vi "Set TimeToPlot.vi"(8 "error in (no error)":errorcluster, 10 "Time to Plot":dbl=1800.0 format="%<%H:%M:%S>t", 11 "BluePlotHandle in":refnum<class "RocketPlotHandle.lvclass">) -> (0 "error out":errorcluster, 3 "BluePlotHandle out":refnum<class "RocketPlotHandle.lvclass">)   [LabVIEW 2021, in "RocketPlotHandle.lvclass"]
doc: "Load plot configuration into the attached plot instance.\n\nNote that this will load ALL plot settings from the input \"plot config\" cluster input.\nThere is no mechanism for specifying only a subset of these settings to be loaded.\nIt's all or nothin'\n\nIf you ever needed to modify/load only 1 aspect of a plot, then I recommend:\n- perform \"get plot config\"\n- perform in-place modification of the plot config cluster to adjust what you want to specifically change\n- perform \"load plot config\""
uses:
  RocketPlotHandle.lvclass
  RocketPlotHandle.lvclass/RocketPlotHandle.ctl
  TypeDefs/plot handle queue data.ctl
  TypeDefs/Plot QSM action.ctl
  RocketPlot.lvlib
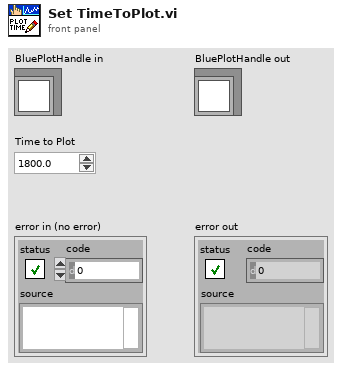
[diagram p1: front panel]
types:
  T1 = typedef "RocketPlot.lvlib/Plot QSM action.ctl" = enum16{"Get Config", "Load Config", "Set TimeToPlot", "Clear Config"}
  T2 = typedef "RocketPlot.lvlib/plot handle queue data.ctl" = cluster{"action":T1, "data":variant}
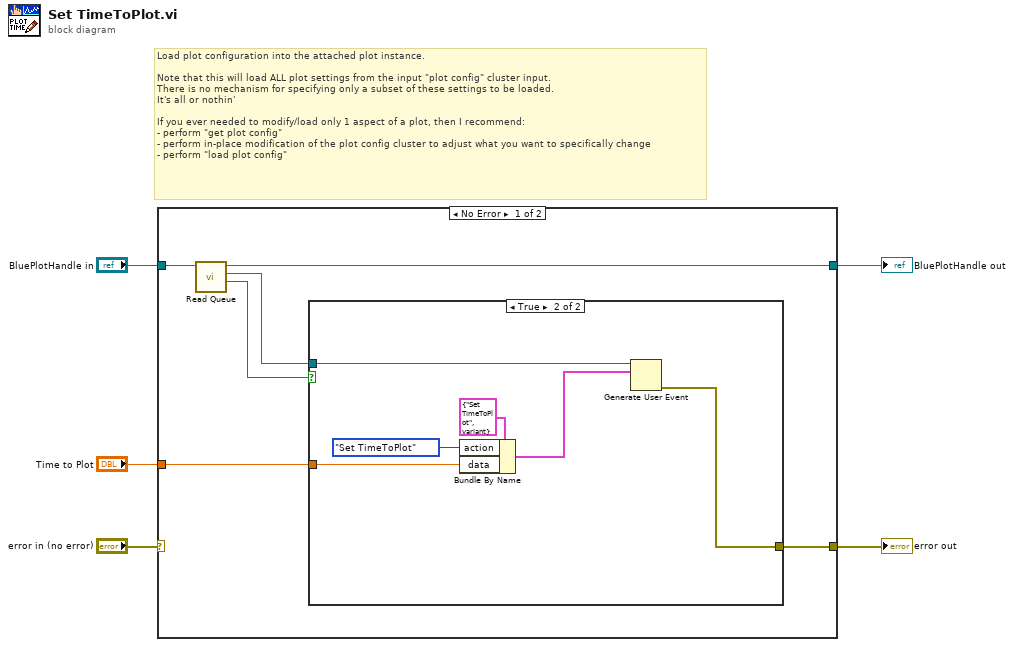
[diagram p0: block diagram]
diagram:
  # "Load plot configuration into the attached plot instance.\n\nNote that this will load ALL plot settings from the input \"plot config\" cluster input.\nThere is no mechanism for specifying only a subset of these settings to be loaded.\nIt's all or nothin'\n\nIf you ever needed to modify/load only 1 aspect of a plot, then I recommend:\n- perform \"get plot config\"\n- perform in-place modification of the plot config cluster to adjust what you want to specifically change\n- perform \"load plot config\""
  n1 = case shown="No Error" "error in (no error)" {
    selector: "error in (no error)" -> [_ w19]
    tunnel: "BluePlotHandle in" -> [w10 w18]
    tunnel: [w7 w19] -> w4
    tunnel: [w8 w18] -> w2
    tunnel: "Time to Plot" -> [w6 _]
    frame No Error {
      n2 = call "Read Queue.vi"("BluePlotHandle in"=w10) -> ("Valid?"=w11:bool, "UE"=w9:refnum<user-event>, "BluePlotHandle out"=w8:refnum<class "RocketPlotHandle.lvclass">)  [unwired: 8 in]
      n3 = case shown="True" w11 {
        tunnel: w9 -> [_ w17]
        tunnel: [_ w13] -> w7
        tunnel: w6 -> [_ w12]
        frame False {
        }
        frame True {
          n4 = Bundle By Name(cluster=T2 {"action"=enum."Set TimeToPlot", "data"=variant} ("element"), "action"=Plot_QSM_action."Set TimeToPlot", "data"=w12) -> (w14:T2)
          n5 = Generate User Event(user event=w17, event data cluster=w14) -> (error out=w13:errorcluster)  [unwired: 2 in, 1 out]
        }
      }
    }
    frame Error {
    }
  }
  "BluePlotHandle out" <- w2
  "error out" <- w4
